vi "LAC initialize.vi"(7 "timeout(ms)":u32, 8 "error in":errorcluster, 9 "data bits (8)":u16, 10 "baud rate":u32, 11 "VISA Refnum in":refnum<visa-resource-name>) -> (0 "error out":errorcluster, 3 "VISA Refnum out":refnum<visa-resource-name>)   [LabVIEW 8.6]
uses:
  <vilib>/Instr/_visa.llb/VISA Configure Serial Port (Instr).vi
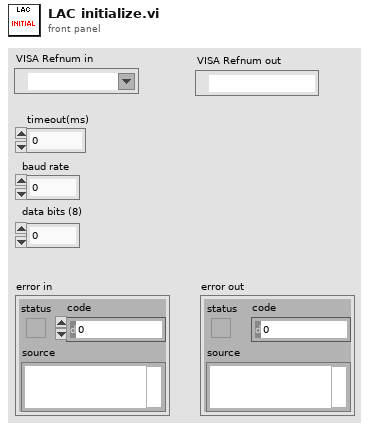
[diagram p1: front panel]
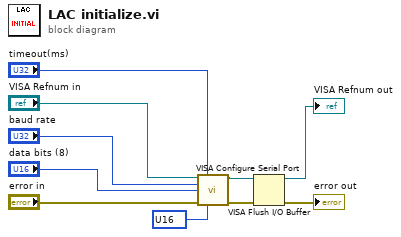
[diagram p0: block diagram]
diagram:
  w10 = u16 ? items=["1.0", "1.5", "2.0"] ("stop bits (10: 1 bit)")
  n1 = call-poly "VISA Configure Serial Port"("VISA resource name"="VISA Refnum in", "timeout (10sec)"="timeout(ms)", "baud rate (9600)"="baud rate", "data bits (8)"="data bits (8)", "error in (no error)"="error in", "stop bits (10: 1 bit)"=w10) -> ("VISA resource name out"=w4:refnum<visa-resource-name>, "error out"=w2:errorcluster)  [unwired: 8 in]
  n2 = VISA Flush I/O Buffer(VISA resource name=w4, error in (no error)=w2) -> (VISA resource name out=→"VISA Refnum out":refnum<visa-resource-name>, error out=→"error out":errorcluster)  [unwired: 1 in]
